vi "Send Abs Start Test.vi"(8 "error in (no error)":errorcluster, 10 "Selected Tests":string[](array[string]), 11 "User Interface in":refnum<class "User Interface.lvclass">) -> (0 "error out":errorcluster, 3 "User Interface out":refnum<class "User Interface.lvclass">)   [LabVIEW 2017, in "User Interface.lvlib" / "User Interface.lvclass"]
uses:
  User Interface.lvclass
  C:/Program Files (x86)/National Instruments/LabVIEW 2017/vi.lib/ActorFramework/Actor/Actor.lvclass
  <vilib>/ActorFramework/Actor/Actor.lvclass/Actor.ctl
  User Interface.lvclass/User Interface.ctl
  User Interface Messages/Start Test Msg/Start Test Msg.lvclass/Start Test Msg.ctl
  <vilib>/ActorFramework/Message Enqueuer/Message Enqueuer.lvclass/Message Enqueuer.ctl
  <vilib>/ActorFramework/Message Enqueuer/Enqueue.vi
  User Interface Messages/Start Test Msg/Start Test Msg.lvclass
  C:/Program Files (x86)/National Instruments/LabVIEW 2017/vi.lib/ActorFramework/Message/Message.lvclass
  <vilib>/ActorFramework/Message Priority Queue/Priority Enqueue.vi
  <vilib>/ActorFramework/Actor/Actor.lvclass
panel:
  # "This Method will Send an Abstract Message To Caller to Start the Test"
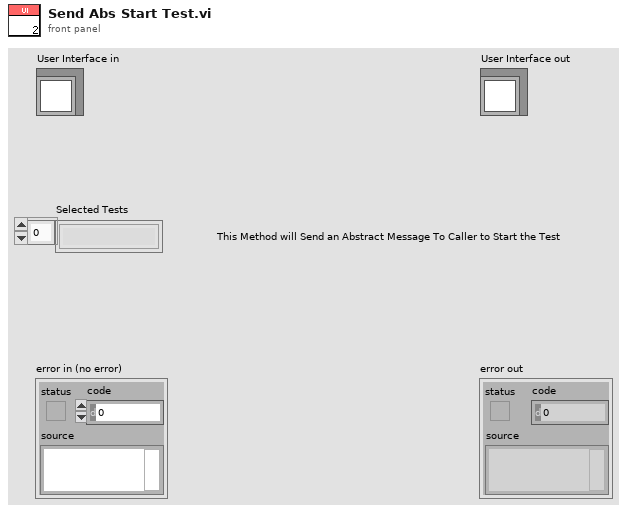
[diagram p1: front panel]
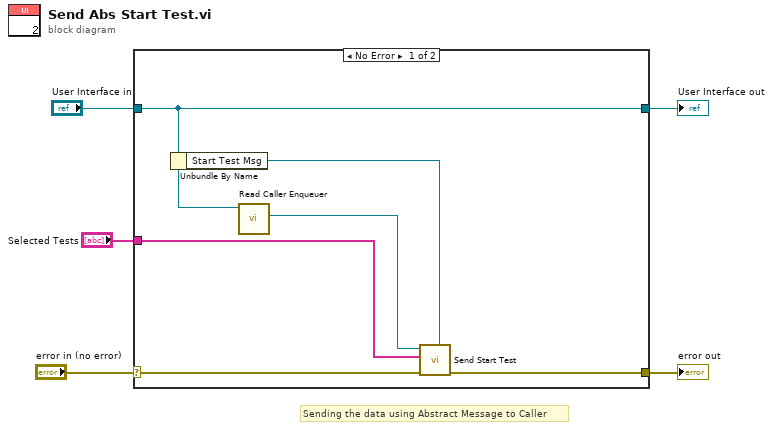
[diagram p0: block diagram]
diagram:
  # "Sending the data using Abstract Message to Caller"
  n1 = case shown="No Error" "error in (no error)" {
    selector: "error in (no error)" -> [w7 w13]
    tunnel: [w6 w13] -> w4
    tunnel: [w11 w12] -> w2
    tunnel: "User Interface in" -> [w11 w12]
    tunnel: "Selected Tests" -> [w8 _]
    frame No Error {
      n2 = Unbundle By Name(w11) -> ("Start Test Msg"=w9:refnum<class "Start Test Msg.lvclass">)
      n3 = call <vilib>:"Read Caller Enqueuer.vi"("Actor"=w11) -> ("Caller Enqueuer"=w10:refnum<class "Message Enqueuer.lvclass">)  [unwired: 10 in]
      n4 = call "Send Start Test.vi"("Message Type"=w9, "error in (no error)"=w7, "Selected Tests"=w8, "Message Enqueuer"=w10) -> ("error out"=w6:errorcluster)  [unwired: 6 in, 1 out]
    }
    frame Error {
    }
  }
  "error out" <- w4
  "User Interface out" <- w2
